vi "Untitled 2.vi"() -> ()   [LabVIEW 2019]
uses:
  CoolProp_advanced.llb/FluidOfInterest.ctl
  CoolProp_advanced.llb/FluidCommon.ctl
  Coolprop_lib.lvlib
panel:
  out "Common Out 3":T1
  out "Common Out 2":T1
  out "Common Out":T1
  in  "Path to CoolProp.dll":path=path "C:/Users/anton/OneDrive - Aarhus universitet/Arbejde/M4INS_F21/Coolprop_simpel/Files/Coolprop_64bit/CoolProp.dll"
  in  "FluidOfInterest":T2="Water"
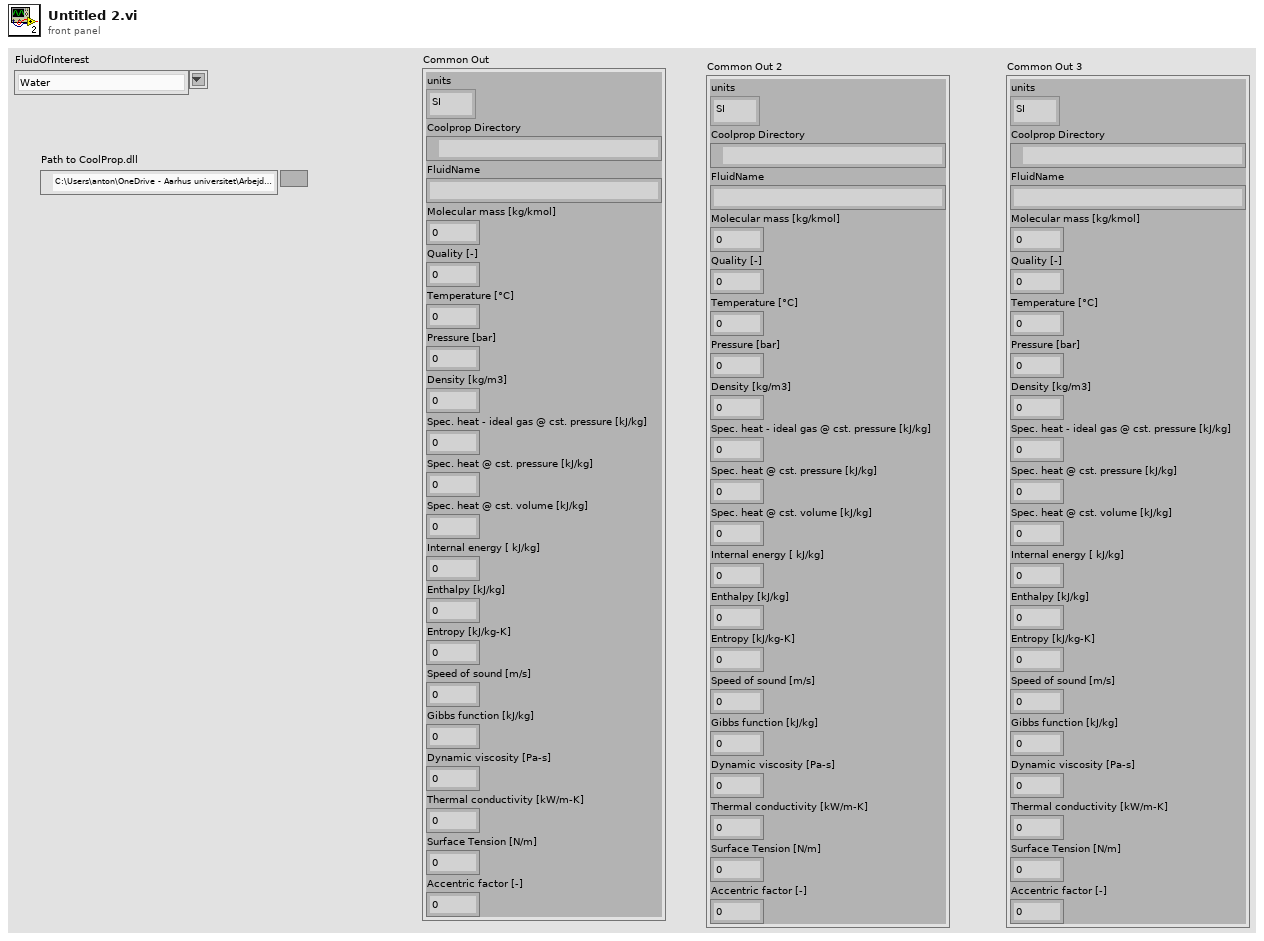
[diagram p1: front panel]
types:
  T1 = typedef "Coolprop_lib.lvlib/FluidCommon.ctl" = cluster{"units":enum16{"SI", "IP"}, "Coolprop Directory":path, "FluidName":string, "Molecular mass [kg/kmol]":dbl, "Quality [-]":dbl, "Temperature [°C]":dbl, "Pressure [bar]":dbl, "Density [kg/m3]":dbl, "Spec. heat - ideal gas @ cst. pressure [kJ/kg]":dbl, "Spec. heat @ cst. pressure [kJ/kg]":dbl, "Spec. heat @ cst. volume [kJ/kg]":dbl, "Internal energy [ kJ/kg]":dbl, "Enthalpy [kJ/kg]":dbl, "Entropy [kJ/kg-K]":dbl, "Speed of sound [m/s]":dbl, "Gibbs function [kJ/kg]":dbl, "Dynamic viscosity [Pa-s]":dbl, "Thermal conductivity [kW/m-K]":dbl, "Surface Tension [N/m]":dbl, "Accentric factor [-]":dbl}
  T2 = typedef "Coolprop_lib.lvlib/FluidOfInterest.ctl" = string
  T3 = enum16{"0", "TP", "TD", "PD", "TQ", "PQ", "HP", "SP", "SH"}
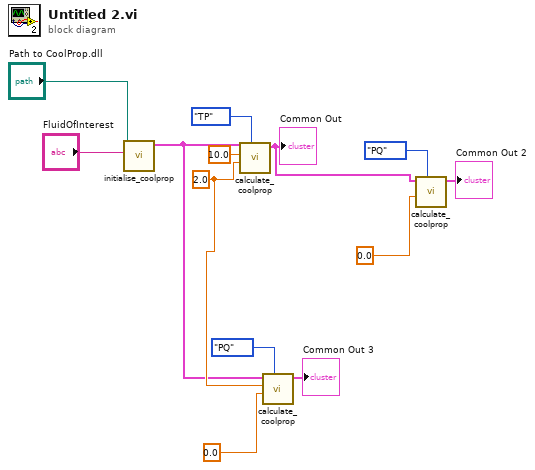
[diagram p0: block diagram]
diagram:
  w2 = 2.0 ("Input_2")
  n1 = call "initialise_coolprop.vi"("Path to CoolProp.dll"="Path to CoolProp.dll", "FluidOfInterest"="FluidOfInterest") -> ("Common Out"=w1:T1)  [unwired: 7 in, 2 out]
  n2 = call "calculate_coolprop.vi"("InputCode"=T3."TP", "Input_2"=w2, "Input_1"=10.0, "Common In"=w1) -> ("Common Out"=w6:T1)  [unwired: 3 in, 1 out]
  "Common Out" <- w6
  n3 = call "calculate_coolprop.vi"("InputCode"=T3."PQ", "Input_2"=0.0, "Input_1"=w2, "Common In"=w1) -> ("Common Out"=→"Common Out 3":T1)  [unwired: 3 in, 1 out]
  n4 = call "calculate_coolprop.vi"("InputCode"=T3."PQ", "Input_2"=0.0, "Common In"=w6) -> ("Common Out"=→"Common Out 2":T1)  [unwired: 4 in, 1 out]
